vi "Create (Ref).vi"(6 "Color (Default)":u32(colorbox)=4547941, 7 "Name":string, 8 "error in (no error)":errorcluster, 9 "Allow Close (T)":bool=TRUE, 10 "VI":refnum<vi>) -> (0 "error out":errorcluster, 3 "PluginGUI out":refnum<class "PluginGUI.lvclass">)   [LabVIEW 2020, in "VolatusGUI.lvlib" / "PluginGUI.lvclass"]
uses:
  PluginGUI.lvclass
  GUI Type.ctl
  PluginGUI.lvclass/PluginGUI.ctl
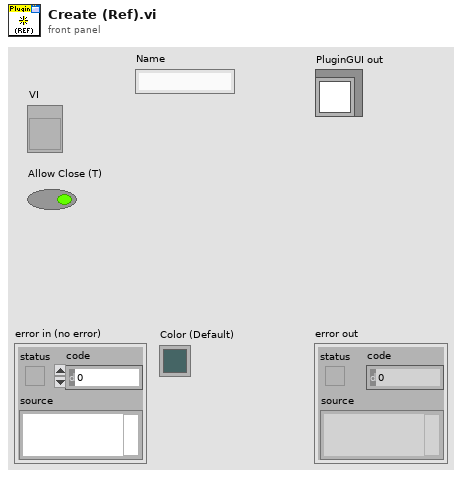
[diagram p1: front panel]
types:
  T1 = typedef "VolatusGUI.lvlib/PluginGUI.lvclass/GUI Type.ctl" = enum16{"Unknown", "Config", "Path", "Ref"}
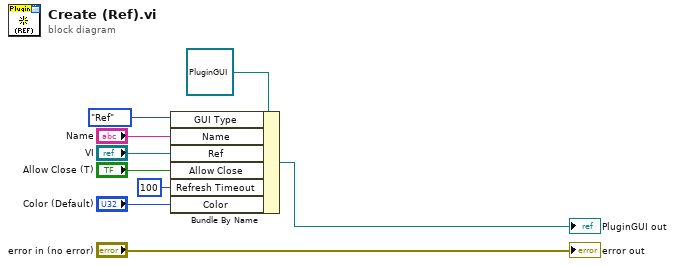
[diagram p0: block diagram]
diagram:
  n1 = Bundle By Name(cluster=refnum<class "PluginGUI.lvclass"> refnum ("PluginGUI in"), "GUI Type"=GUI_Type."Ref", "Name"="Name", "Ref"="VI", "Allow Close"="Allow Close (T)", "Refresh Timeout"=100, "Color"="Color (Default)") -> (→"PluginGUI out":refnum<class "PluginGUI.lvclass">)
  "error out" <- "error in (no error)"
